vi "FSK_Channel.vi"(0 "PathIn":path, 5 "channel_flag":dbl format="%#_13g", 7 "Fs":cdb format="%#_13g", 9 "SendSig":cdb[](array[numeric]) format="%#_13g", 11 "error in (no error)":errorcluster caption="错误输入（无错误）", 12 "簇":T1 {"信噪比(dB)" format="%#_13g"; "P" format="%#_13g"; "F" format="%#_13g"; "T" format="%#_13g"; "A" format="%#_13g"}) -> (4 "PathOut":path, 8 "RecvSig":cdb[](array[numeric]) format="%#_13g", 15 "error out":errorcluster caption="错误输出")   [LabVIEW 2015]
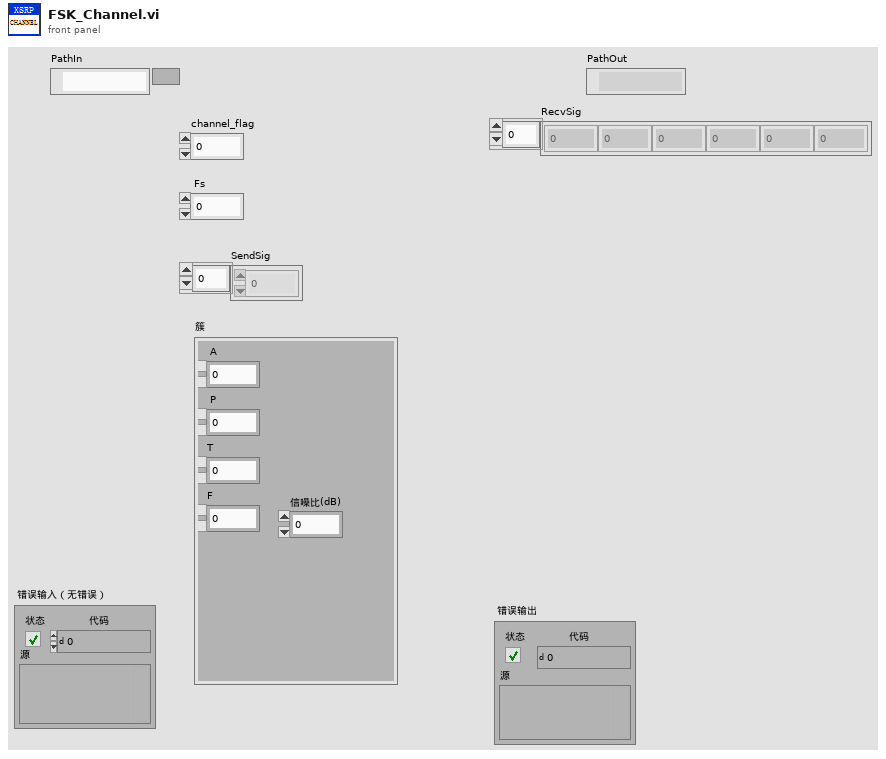
[diagram p1: front panel]
types:
  T1 = cluster{" A":dbl, "T":dbl, "F":dbl, " P":dbl, "信噪比(dB)":dbl}
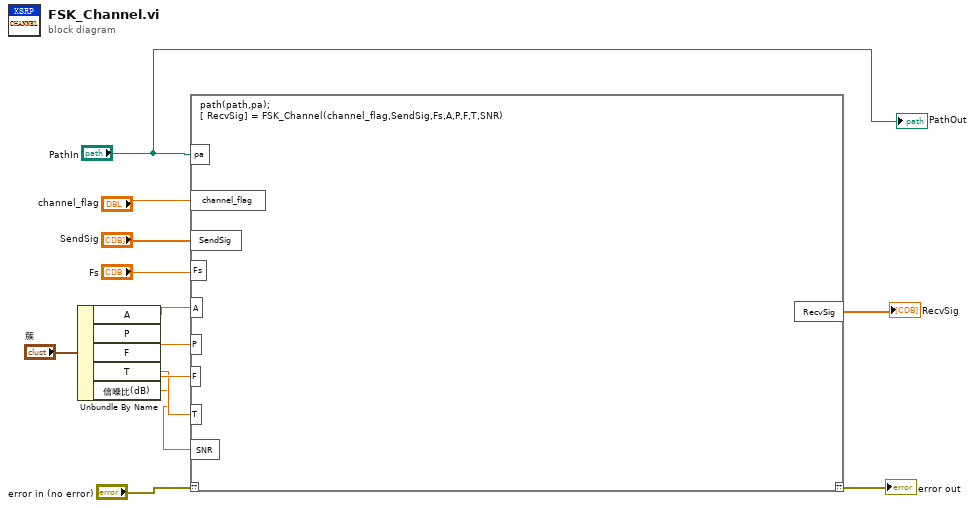
[diagram p0: block diagram]
diagram:
  n1 = Unbundle By Name("簇") -> ("A"=w5:dbl, "P"=w4:dbl, "F"=w3:dbl, "T"=w2:dbl, "信噪比(dB)"=w1:dbl)
  n2 = script code="path(path,pa);\n[ RecvSig] = FSK_Channel(channel_flag,SendSig,Fs,A,P,F,T,SNR)"("??"="error in (no error)", "pa"="PathIn", "channel_flag"="channel_flag", "SendSig"="SendSig", "Fs"="Fs", "A"=w5, "P"=w4, "F"=w3, "T"=w2, "SNR"=w1) -> ("??"=→"error out":errorcluster, "RecvSig"=→"RecvSig":cdb[])
  "PathOut" <- "PathIn"
